vi "Read Roughness.vi"(8 "error in (no error)":errorcluster, 11 "Video Processor in":refnum<class "Video Processor.lvclass">) -> (0 "error out":errorcluster, 2 "Roughness":T1, 3 "Video Processor out":refnum<class "Video Processor.lvclass">)   [LabVIEW 2018, in "Video Processor.lvclass"]
uses:
  Video Processor.lvclass
  Video Processor.lvclass/Video Processor.ctl
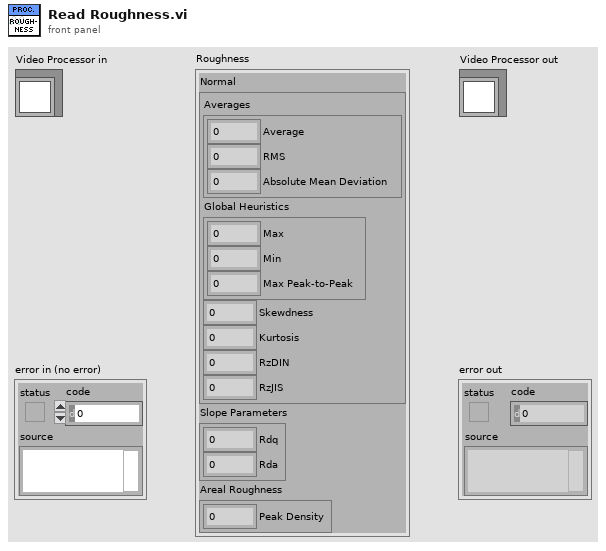
[diagram p1: front panel]
types:
  T1 = cluster{"Normal":cluster{"Averages":cluster{"Average":dbl, "RMS":dbl, "Absolute Mean Deviation":dbl}, "Global Heuristics":cluster{"Max":dbl, "Min":dbl, "Max Peak-to-Peak":dbl}, "Skewdness":dbl, "Kurtosis":dbl, "RzDIN":dbl, "RzJIS":dbl}, "Slope Parameters":cluster{"Rdq":dbl, "Rda":dbl}, "Areal Roughness":cluster{"Peak Density":dbl}}
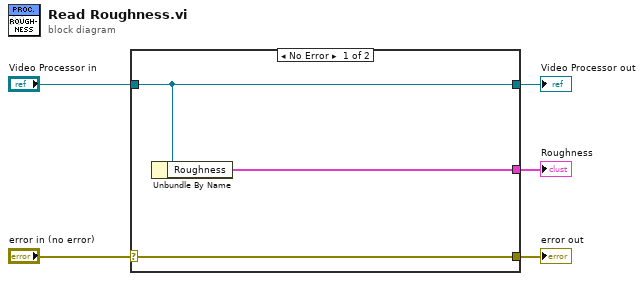
[diagram p0: block diagram]
diagram:
  n1 = case shown="No Error" "error in (no error)" {
    selector: "error in (no error)" -> [w8 w9]
    tunnel: [w8 w9] -> w4
    tunnel: [w7 w10] -> w2
    tunnel: "Video Processor in" -> [w7 w10]
    tunnel: [w6 _] -> w1
    frame No Error {
      n2 = Unbundle By Name(w7) -> ("Roughness"=w6:T1)
    }
    frame Error {
    }
  }
  "error out" <- w4
  "Video Processor out" <- w2
  "Roughness" <- w1
